vi "Set Indicator State By Event.vi"(8 "Value":u16, 9 "New Value?":bool, 10 "No error":bool, 11 "Module Indicator Event":refnum<user-event>) -> ()   [LabVIEW 2020, in "GUI.lvlib" / "GUI.lvclass"]
uses:
  GUI.lvclass
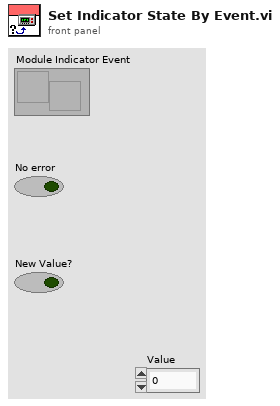
[diagram p1: front panel]
types:
  T1 = cluster{"Boolean 1":bool, "Boolean 2":bool, "Boolean 3":bool, "Boolean 4":bool, "Boolean 5":bool, "Boolean 6":bool, "Boolean 7":bool, "Boolean 8":bool, "Boolean 9":bool, "Boolean 10":bool}
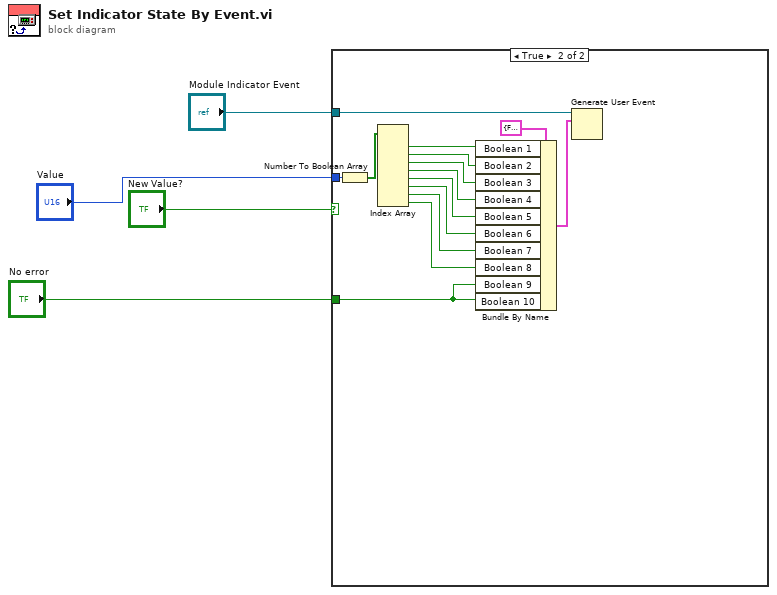
[diagram p0: block diagram]
diagram:
  n1 = case shown="True" "New Value?" {
    tunnel: "Module Indicator Event" -> [_ w18]
    tunnel: "Value" -> [_ w17]
    tunnel: "No error" -> [_ w6]
    frame False {
    }
    frame True {
      n2 = Number To Boolean Array(number=w17) -> (Boolean array=w15:bool[])
      n3 = Index Array(array=w15) -> (element #1=w14:bool, element #2=w13:bool, element #3=w12:bool, element #4=w11:bool, element #5=w10:bool, element #6=w9:bool, element #7=w8:bool, element #8=w7:bool)  [unwired: 8 in]
      n4 = Bundle By Name(cluster=T1 {"Boolean 1"=FALSE, "Boolean 2"=FALSE, "Boolean 3"=FALSE, "Boolean 4"=FALSE, "Boolean 5"=FALSE, "Boolean 6"=FALSE, "Boolean 7"=FALSE, "Boolean 8"=FALSE, "Boolean 9"=FALSE, "Boolean 10"=FALSE} ("event data"), "Boolean 1"=w14, "Boolean 2"=w13, "Boolean 3"=w12, "Boolean 4"=w11, "Boolean 5"=w10, "Boolean 6"=w9, "Boolean 7"=w8, "Boolean 8"=w7, "Boolean 9"=w6, "Boolean 10"=w6) -> (w16:T1)
      n5 = Generate User Event(user event=w18, event data cluster=w16) -> ()  [unwired: 2 in, 2 out]
    }
  }
